vi "TCP Errors conversion.vi"(8 "error in (no error)":errorcluster, 11 "TCP Listener in":refnum<class "TCP Listener.lvclass">) -> (0 "error out":errorcluster, 3 "TCP Listener out":refnum<class "TCP Listener.lvclass">)   [LabVIEW 2026, in "TALOS.lvlib" / "TCP Listener.lvlib" / "TCP Listener.lvclass"]
uses:
  TCP Listener.lvclass
  TCP Listener.lvclass/TCP Listener.ctl
  Ancestor/Ancestor/Ancestor.lvclass/Ancestor.ctl
  Support VIs/Generate Error.vi
  FGV/Error Memory/Get Error Description.vi
  Support VIs/Get PC name.vi
  Ancestor/Ancestor/Read ID.vi
  Support VIs/Get Class Name.vi
  FGV/Error Memory/Error Memory Core.vi
  <vilib>/AdvancedString/Delimited String to 1D String Array.vi
  <vilib>/AdvancedString/Delimited String to 1D String Array (string).vi
  Support VIs/Circus Root Path.vi
  FGV/Error Memory/Error Crt Lvl checker.vi
  FGV/Error Memory/Error Memory Core.vi/40c8088d-b597-4017-91af-faa98e00292e.vi
  FGV/Error Memory/Error Memory Core.vi/d4a3ab98-063c-4e44-b43d-fbdcfe6c2be2.vi
  Support VIs/Global Memory.vi
  <vilib>/Utility/LVClass/Get LV Class Name.vi
  Support VIs/Is in Packed Library.vi
  Support VIs/TALOS Root path.vi
  Support VIs/Read CSV worksheet.vi
  Support VIs/Global Constants.vi
  <vilib>/Utility/error.llb/General Error Handler.vi
  Support VIs/Error Log.vi
  Ancestor/Ancestor/Ancestor.lvclass
  <vilib>/Comparison/Equal/Equal Functor/Equal Functor.lvclass
  TALOS.lvlib
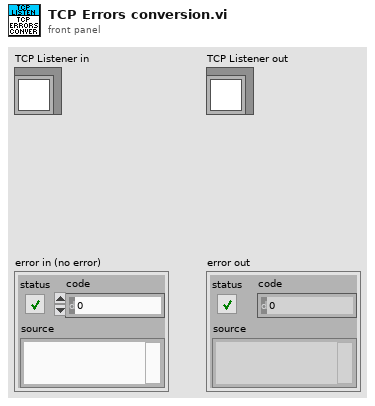
[diagram p1: front panel]
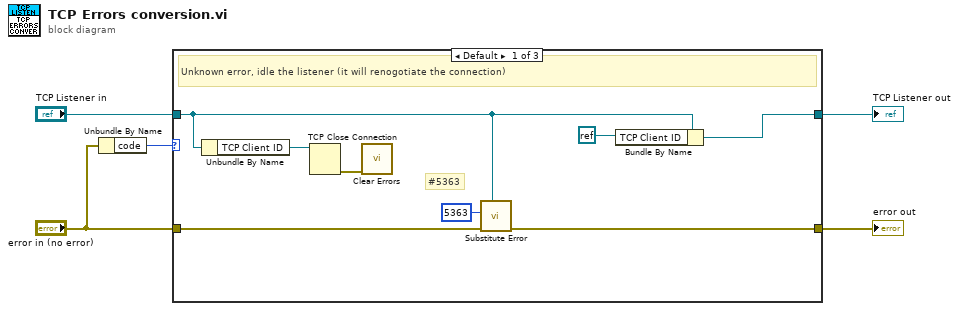
[diagram p0: block diagram]
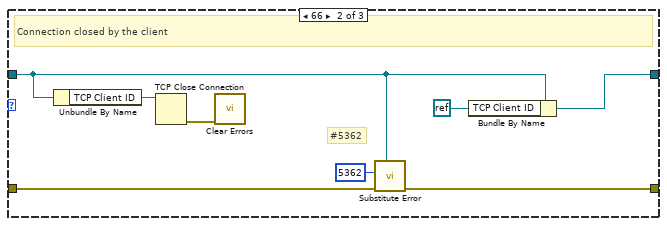
[diagram p2: hidden frame]
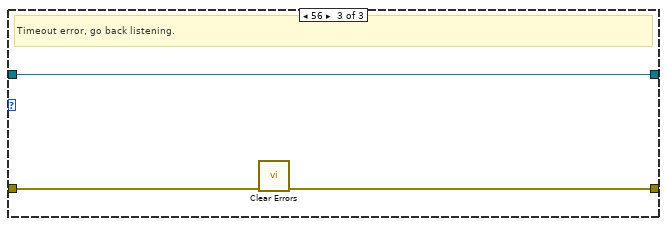
[diagram p3: hidden frame]
diagram:
  n1 = Unbundle By Name("error in (no error)") -> ("code"=w1:i32)
  n2 = case shown="Default" w1 {
    tunnel: [w12 w16 w22] -> w4
    tunnel: "error in (no error)" -> [w13 w21 w23]
    tunnel: "TCP Listener in" -> [w7 w15 w24]
    tunnel: [w8 w18 w24] -> w5
    frame Default {
      # "#5363"
      # "Unknown error, idle the listener (it will renogotiate the connection)"
      n3 = Unbundle By Name(w7) -> ("TCP Client ID"=w6:refnum<k5>)
      n4 = TCP Close Connection(connection ID=w6) -> (error out=w10:errorcluster)  [unwired: 2 in, 1 out]
      n5 = call <vilib>:"Clear Errors.vi"("error in (no error)"=w10) -> ()  [unwired: 5 in, 2 out]
      n6 = call "Substitute Error.vi"("LabVIEW Object"=w7, "error in (no error)"=w13, "Error Code"=5363) -> ("error out"=w12:errorcluster)  [unwired: 8 in]
      n7 = Bundle By Name(cluster=w7, "TCP Client ID"=refnum<k0> refnum) -> (w8:refnum<class "TCP Listener.lvclass">)
    }
    frame 66 {
      # "#5362"
      # "Connection closed by the client"
      n8 = Unbundle By Name(w15) -> ("TCP Client ID"=w14:refnum<k5>)
      n9 = TCP Close Connection(connection ID=w14) -> (error out=w19:errorcluster)  [unwired: 2 in, 1 out]
      n10 = call <vilib>:"Clear Errors.vi"("error in (no error)"=w19) -> ()  [unwired: 5 in, 2 out]
      n11 = call "Substitute Error.vi"("LabVIEW Object"=w15, "error in (no error)"=w21, "Error Code"=5362) -> ("error out"=w16:errorcluster)  [unwired: 8 in]
      n12 = Bundle By Name(cluster=w15, "TCP Client ID"=refnum<k0> refnum) -> (w18:refnum<class "TCP Listener.lvclass">)
    }
    frame 56 {
      # "Timeout error, go back listening."
      n13 = call <vilib>:"Clear Errors.vi"("error in (no error)"=w23) -> ("error out"=w22:errorcluster)  [unwired: 5 in, 1 out]
    }
  }
  "TCP Listener out" <- w5
  "error out" <- w4
